vi "MicroStrain 3DM-GXx Simple Continuous Mode.vi"() -> ()   [LabVIEW 2012]
doc: "Shows how to setup the device and acquire a fixed continuous (streaming) measurement."
uses:
  <instrlib>/MicroStrain 3DM-GXx/Public/Data/Parse Message VIs/Parse (Euler Angles).vi
  <instrlib>/MicroStrain 3DM-GXx/MicroStrain 3DM-GXx.lvlib
panel:
  out "Roll (Degrees)":sgl
  out "Pitch (Degrees)":sgl
  out "Yaw (Degrees)":sgl
  out "Euler Angle Timer":u32
  in  "Sample Rate (100 Hz)":u16=100 min=1 max=300
  in  "VISA resource name":refnum<visa-resource-name>
  in  "Measurement Type":u16(ring)=5 items=["Euler Angles"=5]
  out "Pitch Gauge (Degrees)":dbl(slide) scale=-90.0..90.0
  out "Yaw Gauge (Degrees)":dbl(knob) scale=-180.0..180.0
  out "Roll Gauge (Degrees)":dbl(knob) scale=-180.0..180.0
  in  "Stop Continuous Measurement":bool
  # "This VI demonstrates the procedure for a simiple continuously streaming measurement.  \nThe measurement type has been limited to Euler Angles for simplicity."
  # "(c) 2009 - 2011 National Instruments.  ALL RIGHTS RESERVED."
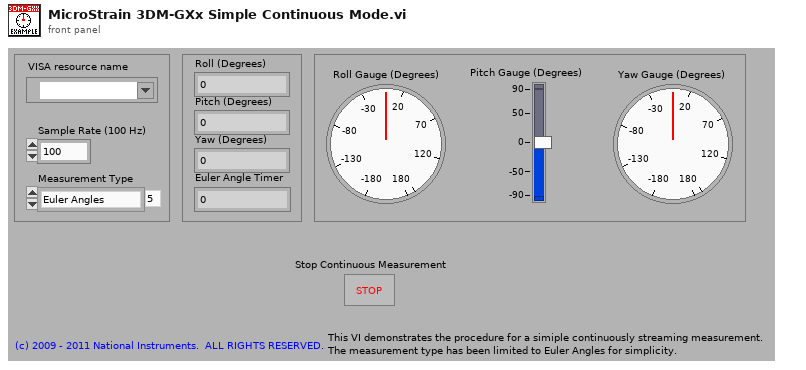
[diagram p1: front panel]
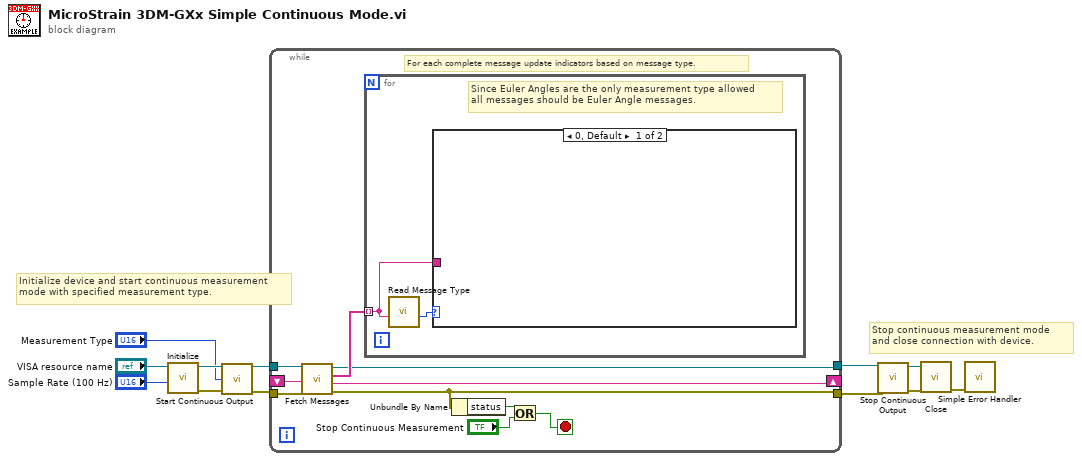
[diagram p0: block diagram]
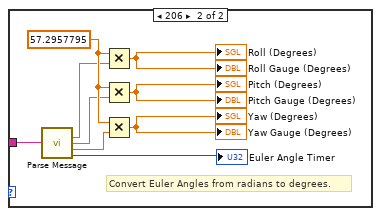
[diagram p2: hidden frame]
diagram:
  # "Stop continuous measurement mode \nand close connection with device."
  # "Initialize device and start continuous measurement \nmode with specified measurement type."
  n1 = call <instrlib>:"Initialize.vi"("Sample Rate (100 Hz)"="Sample Rate (100 Hz)", "VISA resource name"="VISA resource name") -> ("error out"=w11:errorcluster, "VISA resource name out"=w12:refnum<visa-resource-name>)  [unwired: 8 in]
  n2 = call <instrlib>:"Start Continuous Output.vi"("VISA resource name"=w12, "Continuous Measurement Type (Raw Accelerometer and Angular Rate)"="Measurement Type", "error in (no error)"=w11) -> ("VISA resource name out"=w7:refnum<visa-resource-name>, "error out"=w6:errorcluster)  [unwired: 11 in]
  n3 = while {
    tunnel: w7 -> [w22]
    tunnel: w6 -> [w21]
    shift-right: [w19] -> _
    shift-left: _ -> [w20]
    tunnel: [w17] -> w5
    tunnel: [w16] -> w4
    stop <- w13 stop-if-true
    # "For each complete message update indicators based on message type."
    n4 = call <instrlib>:"Fetch Messages.vi"("error in (no error)"=w21, "Remainder In"=w20, "VISA resource name"=w22) -> ("error out"=w16:errorcluster, "Remainder Out"=w19:string, "Complete Messages"=w18:string[], "VISA resource name out"=w17:refnum<visa-resource-name>)  [unwired: 5 in]
    n5 = for {
      tunnel: w18 -> [w23] mode=indexing
      # "Since Euler Angles are the only measurement type allowed \nall messages should be Euler Angle messages."
      n6 = call <instrlib>:"Read Message Type.vi"("Message"=w23) -> ("Ring"=w24:u16)  [unwired: 10 in]
      n7 = case shown="0, Default" w24 {
        tunnel: w23 -> [_ w33]
        frame 0, Default {
        }
        frame 206 {
          w31 = 57.2957795 ("x")
          # "Convert Euler Angles from radians to degrees."
          n8 = call-poly <instrlib>:"Parse Message.vi"("Message In"=w33) -> ("Roll"=w30:sgl, "Pitch"=w29:sgl, "Yaw"=w28:sgl, "Timer"=→"Euler Angle Timer":u32)  [unwired: 11 in]
          n9 = Multiply(x=w31, y=w30) -> (x*y=→"Roll (Degrees)" →"Roll Gauge (Degrees)":dbl)
          n10 = Multiply(x=w31, y=w29) -> (x*y=→"Pitch (Degrees)" →"Pitch Gauge (Degrees)":dbl)
          n11 = Multiply(x=w31, y=w28) -> (x*y=→"Yaw (Degrees)" →"Yaw Gauge (Degrees)":dbl)
        }
      }
    }
    n12 = Unbundle By Name(w16) -> ("status"=w15:bool)
    n13 = Or(x=w15, y="Stop Continuous Measurement") -> (x .or. y?=w13:bool)
  }
  n14 = call <instrlib>:"Stop Continuous Output.vi"("error in (no error)"=w4, "VISA resource name"=w5) -> ("error out"=w3:errorcluster, "VISA resource name out"=w2:refnum<visa-resource-name>)  [unwired: 8 in]
  n15 = call <instrlib>:"Close.vi"("error in (no error)"=w3, "VISA resource name"=w2) -> ("error out"=w1:errorcluster)  [unwired: 9 in]
  n16 = call <vilib>:"Simple Error Handler.vi"("error in (no error)"=w1) -> ()  [unwired: 4 in, 5 out]
